vi "TcA02-007_AttributesCanBeUnlockedWithoutBeingModified.vi"(1 "Input buffer":T3="1", 3 "Invocation info":T2, 5 "error in (no error)":errorcluster, 6 "Add log to result?":bool) -> (16 "Test Data":T1 {"Numeric Measurement" format="%.2f"}, 19 "error out":errorcluster)   [LabVIEW 2020]
doc: "Test case template."
uses:
  Shared/Support_InputBuffer.ctl
  Shared/Support_InvocationInfo.ctl
  Shared/Support_TestData.ctl
  TestClasses/G#SubClass2_class/G#SubClass2.lvclass
  TestClasses/G#BaseClass2_class/G#BaseClass2.lvclass
  <vilib>/addons/_AddQ/G#Object/G#Object.lvclass
panel:
  in  "Test name":string="TcA02-007 Attributes can be unlocked without being modified"
  out "Test result":bool
  out "Result":string
  # "Verify that object attributes can be unlocked without being\nmodified if an error occurs while modifying or forced to be unlocked."
  # "Sub test case"
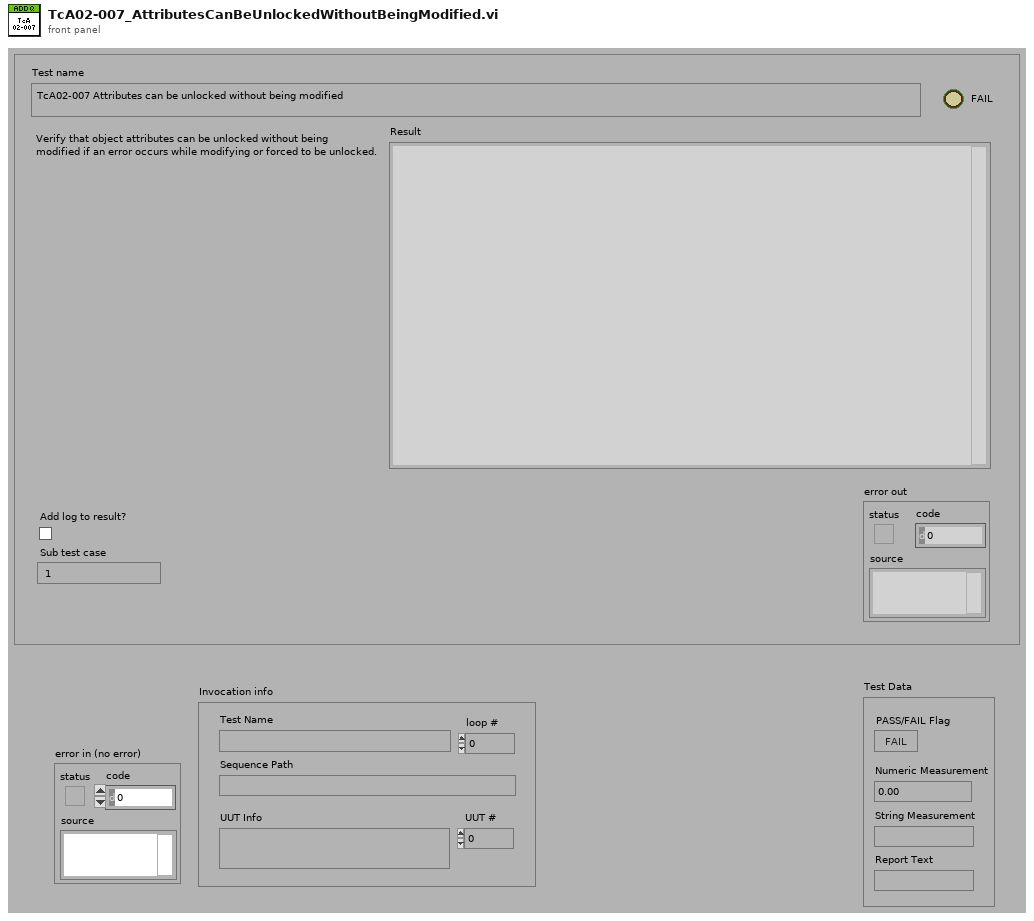
[diagram p1: front panel]
types:
  T1 = typedef "Support_TestData.ctl" = cluster{"PASS/FAIL Flag":bool, "Numeric Measurement":dbl, "String Measurement":string, "Report Text":string}
  T2 = typedef "Support_InvocationInfo.ctl" = cluster{"UUT #":i32, "loop #":i32, "UUT Info":string, "Test Name":string, "Sequence Path":path}
  T3 = typedef "Support_InputBuffer.ctl" = string
  T4 = typedef "Support_ResultType.ctl" = cluster{"Pass":bool, "Comment":string, "MeasurementValue":dbl}
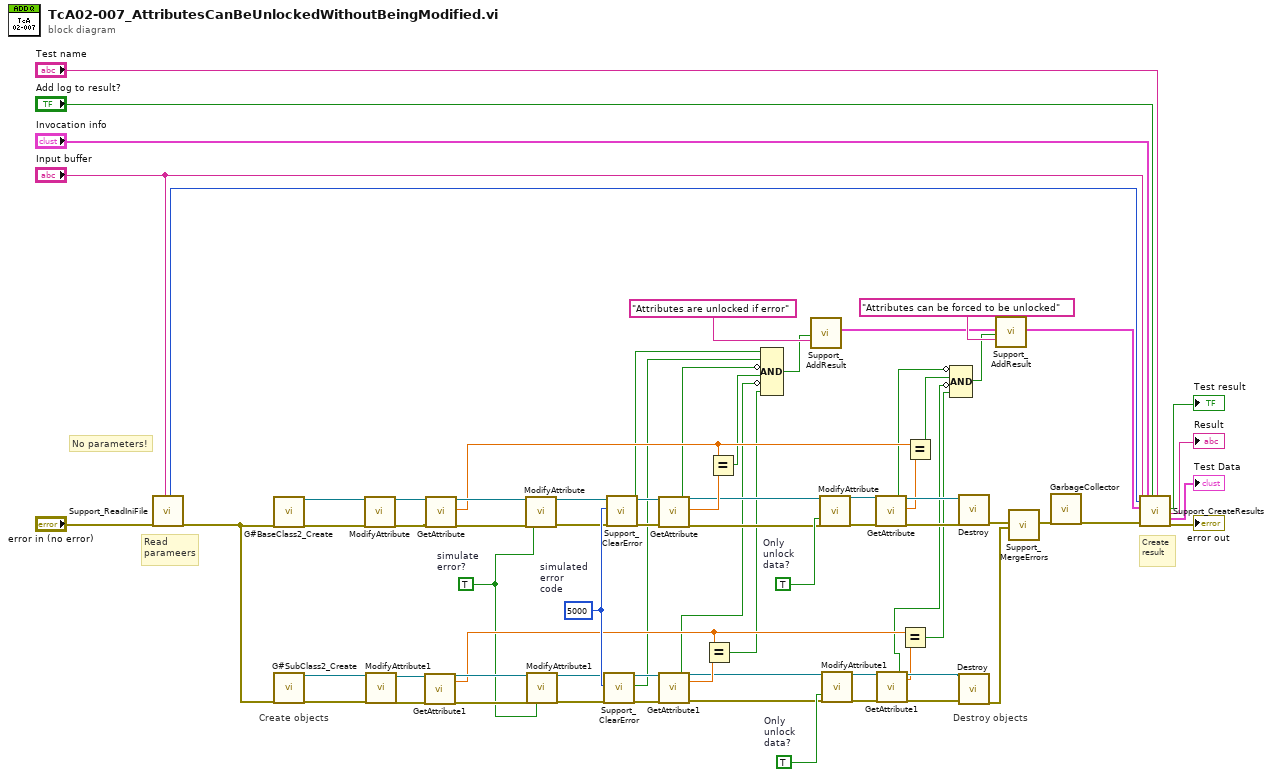
[diagram p0: block diagram]
diagram:
  w29 = TRUE  # Only unlock data?
  w30 = TRUE  # Only unlock data?
  w41 = 5000  # simulated error code
  w3 = TRUE  # simulate error?
  # "Destroy objects"
  # "Create objects"
  # "No parameters!"
  # "Create\nresult"
  # "Read\nparameers"
  n1 = call "Support_ReadIniFile.vi"("error in (no error)"="error in (no error)", "Sub test case"="Input buffer") -> ("Timer start"=w62:u32, "error out"=w61:errorcluster)  [unwired: 10 in, 6 out]
  n2 = call "G#BaseClass2_Create.vi"("error in (no error)"=w61) -> ("reference out"=w59:refnum<class "G#BaseClass2.lvclass">, "error out"=w53:errorcluster)  [unwired: 17 in]
  n3 = call "G#SubClass2_Create.vi"("error in (no error)"=w61) -> ("reference out"=w60:refnum<class "G#SubClass2.lvclass">, "error out"=w52:errorcluster)  [unwired: 17 in]
  n4 = call-dynamic "ModifyAttribute.vi"("reference in"=w59, "error in (no error)"=w53) -> ("reference out"=w49:refnum<class "G#BaseClass2.lvclass">, "error out"=w50:errorcluster)  [unwired: 15 in, 1 out]
  n5 = call-dynamic "ModifyAttribute1.vi"("reference in"=w60, "error in (no error)"=w52) -> ("reference out"=w48:refnum<class "G#SubClass2.lvclass">, "error out"=w51:errorcluster)  [unwired: 15 in, 1 out]
  n6 = call-dynamic "GetAttribute1.vi"("reference in"=w48, "error in (no error)"=w51) -> ("reference out"=w44:refnum<class "G#SubClass2.lvclass">, "Base class.Numeric"=w25:dbl, "error out"=w46:errorcluster)  [unwired: 12 in, 3 out]
  n7 = call-dynamic "GetAttribute.vi"("reference in"=w49, "error in (no error)"=w50) -> ("reference out"=w47:refnum<class "G#BaseClass2.lvclass">, "Numeric"=w27:dbl, "error out"=w45:errorcluster)  [unwired: 13 in, 2 out]
  n8 = call-dynamic "ModifyAttribute.vi"("reference in"=w47, "error in (no error)"=w45, "status"=w3) -> ("reference out"=w16:refnum<class "G#BaseClass2.lvclass">, "error out"=w21:errorcluster)  [unwired: 14 in, 1 out]
  n9 = call-dynamic "ModifyAttribute1.vi"("reference in"=w44, "error in (no error)"=w46, "status"=w3) -> ("reference out"=w17:refnum<class "G#SubClass2.lvclass">, "error out"=w18:errorcluster)  [unwired: 14 in, 1 out]
  n10 = call "Support_ClearError.vi"("code"=w41, "error in (no error)"=w18) -> ("Cleared?"=w1:bool, "error out"=w19:errorcluster)  [unwired: 16 in]
  n11 = call "Support_ClearError.vi"("code"=w41, "error in (no error)"=w21) -> ("Cleared?"=w2:bool, "error out"=w20:errorcluster)  [unwired: 16 in]
  n12 = call-dynamic "GetAttribute.vi"("reference in"=w16, "error in (no error)"=w20) -> ("Locked"=w7:bool, "reference out"=w39:refnum<class "G#BaseClass2.lvclass">, "Numeric"=w43:dbl, "error out"=w15:errorcluster)  [unwired: 13 in, 1 out]
  n13 = call-dynamic "GetAttribute1.vi"("reference in"=w17, "error in (no error)"=w19) -> ("Locked"=w6:bool, "reference out"=w33:refnum<class "G#SubClass2.lvclass">, "Base class.Numeric"=w42:dbl, "error out"=w14:errorcluster)  [unwired: 12 in, 2 out]
  n14 = Equal?(x=w25, y=w42) -> (x = y?=w12:bool)
  n15 = Equal?(x=w27, y=w43) -> (x = y?=w13:bool)
  n16 = Compound Arithmetic op=AND(w2, w1, invert w7, w13, invert w6, w12) -> (w11:bool)
  n17 = call "Support_AddResult.vi"("Pass"=w11, "Comment"="Attributes are unlocked if error") -> ("Results out"=w23:T4[])  [unwired: 17 in]
  n18 = call-dynamic "ModifyAttribute.vi"("reference in"=w39, "Only unlock data? (F)"=w30, "error in (no error)"=w15) -> ("reference out"=w38:refnum<class "G#BaseClass2.lvclass">, "error out"=w40:errorcluster)  [unwired: 14 in, 1 out]
  n19 = call-dynamic "ModifyAttribute1.vi"("reference in"=w33, "Only unlock data? (F)"=w29, "error in (no error)"=w14) -> ("reference out"=w32:refnum<class "G#SubClass2.lvclass">, "error out"=w35:errorcluster)  [unwired: 14 in, 1 out]
  n20 = call-dynamic "GetAttribute.vi"("reference in"=w38, "error in (no error)"=w40) -> ("Locked"=w4:bool, "reference out"=w37:refnum<class "G#BaseClass2.lvclass">, "Numeric"=w28:dbl, "error out"=w36:errorcluster)  [unwired: 13 in, 1 out]
  n21 = call-dynamic "GetAttribute1.vi"("reference in"=w32, "error in (no error)"=w35) -> ("Locked"=w5:bool, "reference out"=w31:refnum<class "G#SubClass2.lvclass">, "Base class.Numeric"=w26:dbl, "error out"=w34:errorcluster)  [unwired: 12 in, 2 out]
  n22 = Equal?(x=w25, y=w26) -> (x = y?=w9:bool)
  n23 = Equal?(x=w27, y=w28) -> (x = y?=w10:bool)
  n24 = Compound Arithmetic op=AND(invert w4, w10, invert w5, w9) -> (w8:bool)
  n25 = call-dynamic "Destroy.vi"("reference in"=w37, "error in (no error)"=w36) -> ("error out"=w55:errorcluster)  [unwired: 16 in, 1 out]
  n26 = call-dynamic "Destroy.vi"("reference in"=w31, "error in (no error)"=w34) -> ("error out"=w54:errorcluster)  [unwired: 16 in, 1 out]
  n27 = call "Support_AddResult.vi"("Results in"=w23, "Pass"=w8, "Comment"="Attributes can be forced to be unlocked") -> ("Results out"=w22:T4[])  [unwired: 16 in]
  n28 = call "Support_MergeErrors.vi"("error in 1"=w55, "error in 2"=w54) -> ("error out"=w58:errorcluster)  [unwired: 16 in, 1 out]
  n29 = call <vilib>:"GarbageCollector.vi"("error in (no error)"=w58) -> ("error out"=w57:errorcluster)  [unwired: 16 in, 2 out]
  n30 = call "Support_CreateResults.vi"("Sub test case"="Input buffer", "Timer start"=w62, "Results"=w22, "error in (no error)"=w57, "Invocation info"="Invocation info", "Add log to result?"="Add log to result?", "Test name"="Test name") -> ("Pass/fail flag"=→"Test result":bool, "Result"=→"Result":string, "Test Data"=→"Test Data":T1, "error out"=→"error out":errorcluster)  [unwired: 9 in]
